vi "4.1.vi"() -> ()   [LabVIEW 2016]
panel:
  out "温度计":dbl(slide) scale=0.0..100.0
  out "波形图表":dbl(graph)
  out "平均值":dbl
  out "最小值":dbl
  out "最大值":dbl
  out "波形图":dbl[](graph)
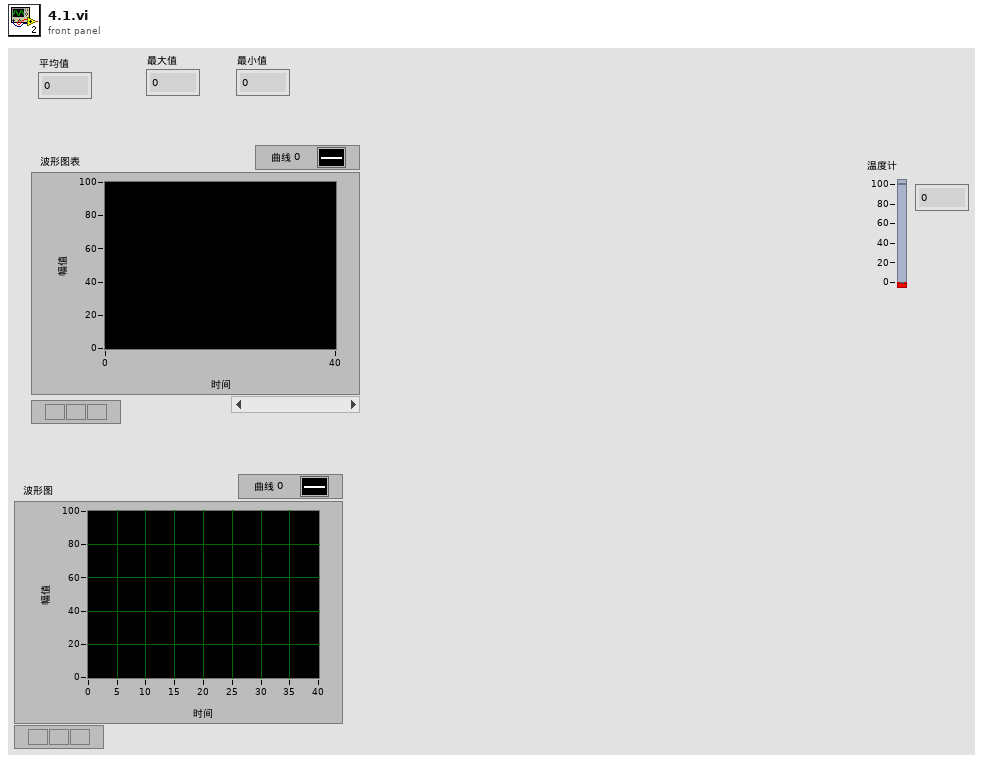
[diagram p1: front panel]
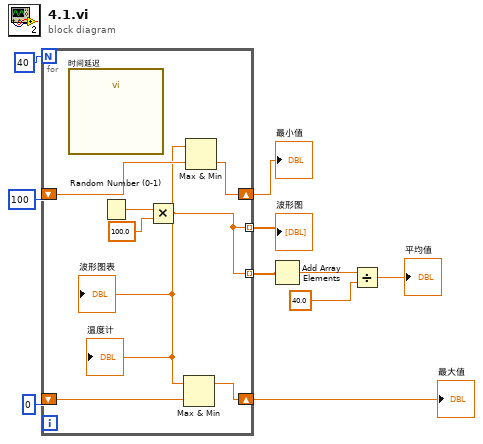
[diagram p0: block diagram]
diagram:
  n1 = for {
    N: 40 -> [_]
    tunnel: [w11] -> w10 mode=indexing
    shift-right: [w16] -> w8
    shift-left: 0 -> [w17]
    shift-right: [w14] -> w6
    shift-left: 100 -> [w15]
    tunnel: [w11] -> w4 mode=indexing
    n2 = call "时间延迟"() -> ()  [unwired: 11 in, 1 out]
    n3 = Random Number (0-1)() -> (number: 0 to 1=w13:dbl)
    n4 = Multiply(x=w13, y=100.0) -> (x*y=w11:dbl)
    "波形图表" <- w11
    "温度计" <- w11
    n5 = Max & Min(x=w11, y=w17) -> (max(x,y)=w16:dbl)  [unwired: 1 out]
    n6 = Max & Min(x=w11, y=w15) -> (min(x,y)=w14:dbl)  [unwired: 1 out]
  }
  "波形图" <- w10
  "最大值" <- w8
  "最小值" <- w6
  n7 = Add Array Elements(numeric array=w4) -> (sum=w3:dbl)
  n8 = Divide(x=w3, y=40.0) -> (x/y=→"平均值":dbl)
